vi "GetPixelData16.vi"(1 "Input buffer":u8[](array[numeric]), 2 "Output buffer in":u16[](array[numeric]), 3 "Pixel Encoding":string, 4 "Stride":i64, 5 "error in (no error)":errorcluster, 7 "Width":i64, 9 "Height":i64) -> (14 "Status":i32, 16 "Output buffer out":u16[](array[numeric]), 19 "error out":errorcluster)   [LabVIEW 2019]
doc: "Get Pixel Data 16\n\nOutput:\n I32 Status\n U16[] Output buffer out\n\nInput:\n U8 Input buffer\n U16[] Output buffer in\n I64 Width\n I64 Height\n I64 Stride\n String Pixel Encoding\n\n\nThis function converts and array of bytes into an array of 16bit pixels."
uses:
  atunpackera.dll
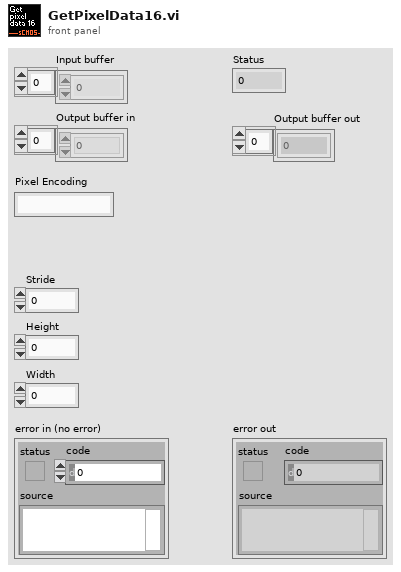
[diagram p1: front panel]
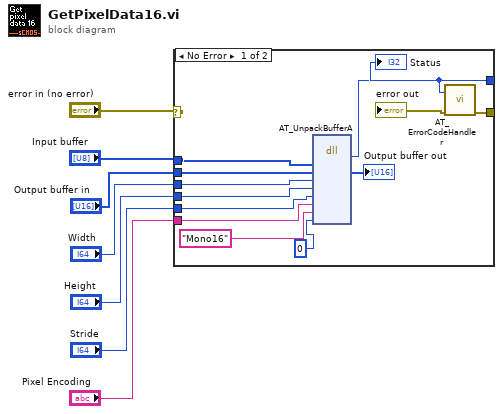
[diagram p0: block diagram]
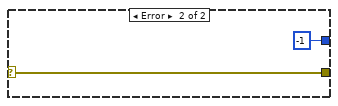
[diagram p2: hidden frame]
diagram:
  n1 = case shown="No Error" "error in (no error)" {
    selector: "error in (no error)" -> [_ w22]
    tunnel: [w12 -1 ("Status")] -> w8
    tunnel: "Width" -> [w19 _]
    tunnel: "Height" -> [w18 _]
    tunnel: "Stride" -> [w17 _]
    tunnel: "Pixel Encoding" -> [w16 _]
    tunnel: "Input buffer" -> [w15 _]
    tunnel: "Output buffer in" -> [w14 _]
    tunnel: [w13 w22] -> w1
    frame No Error {
      n2 = dll-call lib="atunpackera.dll" fn="AT_UnpackBufferA"("Input Buffer"=w15, "Output Buffer"=w14, "Width"=w19, "Height"=w18, "Stride"=w17, "Input Pixel Encoding"=w16, "Output Pixel Encoding"="Mono16", "Number Threads"=i64 0 ("Image size in bytes")) -> ("Status"=w12:i32, "Output Buffer"=→"Output buffer out":u16[])  [unwired: 10 in, 2 out]
      n3 = call <userlib>:"AT_ErrorCodeHandler.vi"("Error"=w12) -> ("error out"=w13:errorcluster)  [unwired: 6 in]
    }
    frame Error {
    }
  }
  "error out" <- w1
  "Status" <- w8
